vi "Variant to Connection.vi"(11 "Value Type":T1) -> (3 "Connection Class":variant)   [LabVIEW 2020, in "Parallel Block.lvlib"]
uses:
  Parallel Block.lvlib
  Value Type.ctl
  Connection/Connection.lvclass
  Bool Connection/Bool Connection.lvclass
  U8 Connection/U8 Connection.lvclass
  U16 Connection/U16 Connection.lvclass
  U32 Connection/U32 Connection.lvclass
  U64 Connection/U64 Connection.lvclass
  I8 Connection/I8 Connection.lvclass
  I16 Connection/I16 Connection.lvclass
  I32 Connection/I32 Connection.lvclass
  I64 Connection/I64 Connection.lvclass
  SGL Connection/SGL Connection.lvclass
  DBL Connection/DBL Connection.lvclass
  CSG Connection/CSG Connection.lvclass
  CDB Connection/CDB Connection.lvclass
  CDBWfm Connection/CDBWfm Connection.lvclass
  DBLWfm Connection/DBLWfm Connection.lvclass
  String Connection/String Connection.lvclass
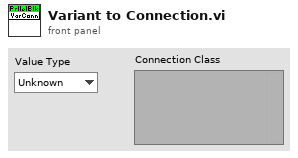
[diagram p1: front panel]
types:
  T1 = typedef "Parallel Block.lvlib/Value Type.ctl" = enum16{"Unknown", "Bool", "U8", "U16", "U32", "U64", "I8", "I16", "I32", "I64", "SGL", "DBL", "CSG", "CDB", "CDBWfm", "String", "DBLWfm"}
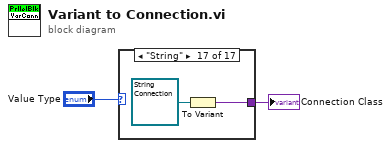
[diagram p0: block diagram]
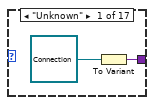
[diagram p2: hidden frame]
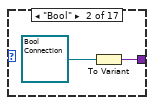
[diagram p3: hidden frame]
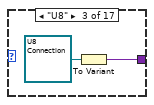
[diagram p4: hidden frame]
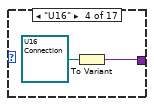
[diagram p5: hidden frame]
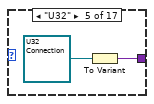
[diagram p6: hidden frame]
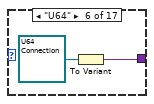
[diagram p7: hidden frame]
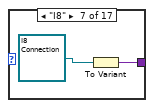
[diagram p8: hidden frame]
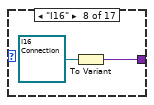
[diagram p9: hidden frame]
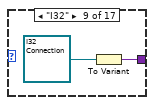
[diagram p10: hidden frame]
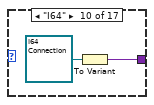
[diagram p11: hidden frame]
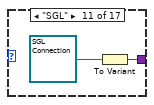
[diagram p12: hidden frame]
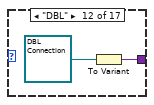
[diagram p13: hidden frame]
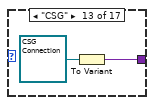
[diagram p14: hidden frame]
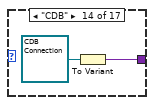
[diagram p15: hidden frame]
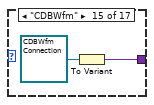
[diagram p16: hidden frame]
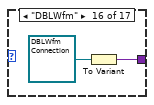
[diagram p17: hidden frame]
diagram:
  n1 = case shown="\"String\"" "Value Type" {
    tunnel: [w3 w5 w7 w9 w11 w13 w15 w17 w19 w21 w24 w25 w27 w29 w31 w33 w35] -> w1
    frame "Unknown" {
      n2 = To Variant(anything=refnum<class "Connection.lvclass"> refnum ("Parallel Block.lvlib:Connection.lvclass")) -> (Variant=w3:variant)
    }
    frame "Bool" {
      n3 = To Variant(anything=refnum<class "Bool Connection.lvclass"> refnum ("Parallel Block.lvlib:Bool Connection.lvclass")) -> (Variant=w5:variant)
    }
    frame "U8" {
      n4 = To Variant(anything=refnum<class "U8 Connection.lvclass"> refnum ("Parallel Block.lvlib:U8 Connection.lvclass")) -> (Variant=w7:variant)
    }
    frame "U16" {
      n5 = To Variant(anything=refnum<class "U16 Connection.lvclass"> refnum ("Parallel Block.lvlib:U16 Connection.lvclass")) -> (Variant=w9:variant)
    }
    frame "U32" {
      n6 = To Variant(anything=refnum<class "U32 Connection.lvclass"> refnum ("Parallel Block.lvlib:U32 Connection.lvclass")) -> (Variant=w11:variant)
    }
    frame "U64" {
      n7 = To Variant(anything=refnum<class "U64 Connection.lvclass"> refnum ("Parallel Block.lvlib:U64 Connection.lvclass")) -> (Variant=w13:variant)
    }
    frame "I8" {
      n8 = To Variant(anything=refnum<class "I8 Connection.lvclass"> refnum ("Parallel Block.lvlib:I8 Connection.lvclass")) -> (Variant=w15:variant)
    }
    frame "I16" {
      n9 = To Variant(anything=refnum<class "I16 Connection.lvclass"> refnum ("Parallel Block.lvlib:I16 Connection.lvclass")) -> (Variant=w17:variant)
    }
    frame "I32" {
      n10 = To Variant(anything=refnum<class "I32 Connection.lvclass"> refnum ("Parallel Block.lvlib:I32 Connection.lvclass")) -> (Variant=w19:variant)
    }
    frame "I64" {
      n11 = To Variant(anything=refnum<class "I64 Connection.lvclass"> refnum ("Parallel Block.lvlib:I64 Connection.lvclass")) -> (Variant=w21:variant)
    }
    frame "SGL" {
      n12 = To Variant(anything=refnum<class "SGL Connection.lvclass"> refnum ("Parallel Block.lvlib:SGL Connection.lvclass")) -> (Variant=w24:variant)
    }
    frame "DBL" {
      n13 = To Variant(anything=refnum<class "DBL Connection.lvclass"> refnum ("Parallel Block.lvlib:DBL Connection.lvclass")) -> (Variant=w25:variant)
    }
    frame "CSG" {
      n14 = To Variant(anything=refnum<class "CSG Connection.lvclass"> refnum ("Parallel Block.lvlib:CSG Connection.lvclass")) -> (Variant=w27:variant)
    }
    frame "CDB" {
      n15 = To Variant(anything=refnum<class "CDB Connection.lvclass"> refnum ("Parallel Block.lvlib:CDB Connection.lvclass")) -> (Variant=w29:variant)
    }
    frame "CDBWfm" {
      n16 = To Variant(anything=refnum<class "CDBWfm Connection.lvclass"> refnum ("Parallel Block.lvlib:CDBWfm Connection.lvclass")) -> (Variant=w31:variant)
    }
    frame "DBLWfm" {
      n17 = To Variant(anything=refnum<class "DBLWfm Connection.lvclass"> refnum ("Parallel Block.lvlib:DBLWfm Connection.lvclass")) -> (Variant=w33:variant)
    }
    frame "String" {
      n18 = To Variant(anything=refnum<class "String Connection.lvclass"> refnum ("Parallel Block.lvlib:String Connection.lvclass")) -> (Variant=w35:variant)
    }
  }
  "Connection Class" <- w1
